vi "Set TWM Processing.vi"(4 "status ref (none)":refnum<vi>, 7 "Measurement properties":T1={"Measurement ID"=enum."1 signal, 1 ADC, 1 PJVS", "Description"="3 phase, 3 ADC, 1 PJVS", "Switching matrix M"=[], "Signal frequency  (Hz)"=50.0, "Maximal signal amplitude (V)"=0.0, "PRs (samples)"=0, "PRe (samples)"=0, "MRs (samples)"=0, "MRe (samples)"=0, "Set PJVS frequency (Hz)"=50.0, "PJVS reference voltages (1 period, V)"=[], "Requested PJVS frequency (Hz)"=50.0, "Requiested PJVS steps"=10, "Sampling f (Hz)"=7000.0, "Trigger mode"=enum."Trigger every MX switch", "Timing matrix (periods)"=[], "Record length (multiples of M)"=1, "Calculated"={"Triggers to next path (line of sequence)"=[], "Record samples"=0, "Sample indexes of switches"=[], "PRs (s)"=0.0, "PRe (s)"=0.0, "MRs (s)"=0.0, "MRe (s)"=0.0, "Trigger frequency  (Hz)"=50.0, "Measurement druation (s)"=0.0, "Samples per step"=0.0, "QPMX Sequence"=[], "PJVS segments frequency (Hz)"=50.0}, "No of required digitizers"=0, "No of required transducers"=0, "Transducer correction files"=[], "Digitizer correction file"=path "", "Algorithm"="TWM-PWRFFT", "plots_level"=1, "calc results"=FALSE, "Calculation mode"=enum."Standard"} {"Requested PJVS frequency (Hz)" format="%#_6p"; "plots_level" max=4 step=1; "Calculated"."Trigger frequency  (Hz)" format="%#_6p"; "Record length (multiples of M)" min=1 step=1; "PJVS reference voltages (1 period, V)" format="%.9g"}, 8 "error in":errorcluster, 11 "handle":i32) -> (0 "error out":errorcluster, 3 "handle out":i32)   [LabVIEW 2020]
doc: "Sets data processing in TWM. Sets algorithm and parameters."
uses:
  Type definitions/Measuement properties.ctl
  Type definitions/Measurement ID.ctl
  Type definitions/Trigger mode.ctl
  Type definitions/Calculation mode.ctl
  external libraries/TWM client/TWM Client Meas Setup.ctl
  external libraries/TWM client/TWM Client Meas Setup Trig.ctl
  external libraries/TWM client/TWM Client Processing Setup.ctl
  external libraries/TWM client/TWM Client.lvlib
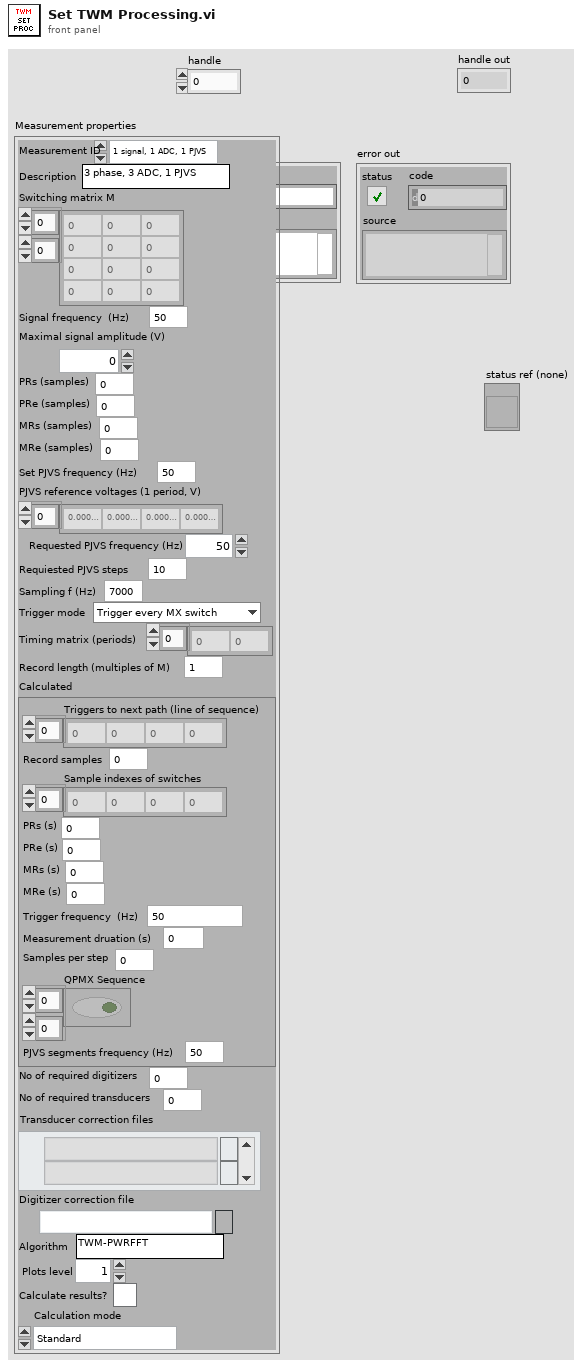
[diagram p1: front panel]
types:
  T1 = typedef "Measuement properties.ctl" = cluster{"Measurement ID":T2, "Description":string, "Switching matrix M":i32[][], "Signal frequency  (Hz)":dbl, "Maximal signal amplitude (V)":dbl, "PRs (samples)":u32, "PRe (samples)":u32, "MRs (samples)":u32, "MRe (samples)":u32, "Set PJVS frequency (Hz)":dbl, "PJVS reference voltages (1 period, V)":dbl[], "Requested PJVS frequency (Hz)":dbl, "Requiested PJVS steps":u32, "Sampling f (Hz)":dbl, "Trigger mode":T3, "Timing matrix (periods)":i32[], "Record length (multiples of M)":u32, "Calculated":cluster{"Triggers to next path (line of sequence)":u32[], "Record samples":u32, "Sample indexes of switches":u32[], "PRs (s)":dbl, "PRe (s)":dbl, "MRs (s)":dbl, "MRe (s)":dbl, "Trigger frequency  (Hz)":dbl, "Measurement druation (s)":dbl, "Samples per step":dbl, "QPMX Sequence":bool[][], "PJVS segments frequency (Hz)":dbl}, "No of required digitizers":u32, "No of required transducers":u32, "Transducer correction files":path[], "Digitizer correction file":path, "Algorithm":string, "plots_level":u32, "calc results":bool, "Calculation mode":T4}
  T2 = typedef "Measurement ID.ctl" = enum16{"Manual setup", "1 signal, 1 ADC, 1 PJVS", "1 phase (U, I), 1 ADC, 1 PJVS", "1 phase (U, I), 2 ADC, 1 PJVS, 4to1", "1 phase (U, I), 2 ADC, 1 PJVS, 2to1", "1 phase (U, I), 3 ADC, 1 PJVS", "3 phases (U1..3, I1..3), 3 ADC, 1 PJVS"}
  T3 = typedef "Trigger mode.ctl" = enum16{"Trigger every MX switch", "Trigger every sample"}
  T4 = typedef "Calculation mode.ctl" = enum16{"Standard", "Only synchronous power"}
  T5 = typedef "TWM Client.lvlib/TWM Client Processing Setup.ctl" = cluster{"calculate":i32, "all cycles at once":bool, "alg. ID":string, "unc mode":string, "mc cycles":i32, "timeout [s]":dbl, "loc [-]":dbl, "valid?":bool, "qwtb params":cluster{"name":string, "data":string[]}[]}
  T6 = typedef "TWM Client.lvlib/TWM Client Meas Setup Trig.ctl" = cluster{"valid?":bool, "coupling (T is DC)":bool, "slope (T is positive)":bool, "source (Immediate)":enum16{"Immediate", "Level", "External"}, "level [V]":dbl, "hysteresis [V]":dbl, "pre-trigger [%]":dbl}
  T7 = typedef "TWM Client.lvlib/TWM Client Meas Setup.ctl" = cluster{"smpl count":i32, "smpl rate [Hz]":dbl, "average":i32, "aperture [s]":dbl, "valid?":bool, "meas fld":path, "sub-records":i32, "ranges [Vpk]":dbl[], "smpl rate - fr [Hz]":dbl, "smpl rate - div":dbl, "smpl rate - mul":dbl, "offsets [V]":dbl[]}
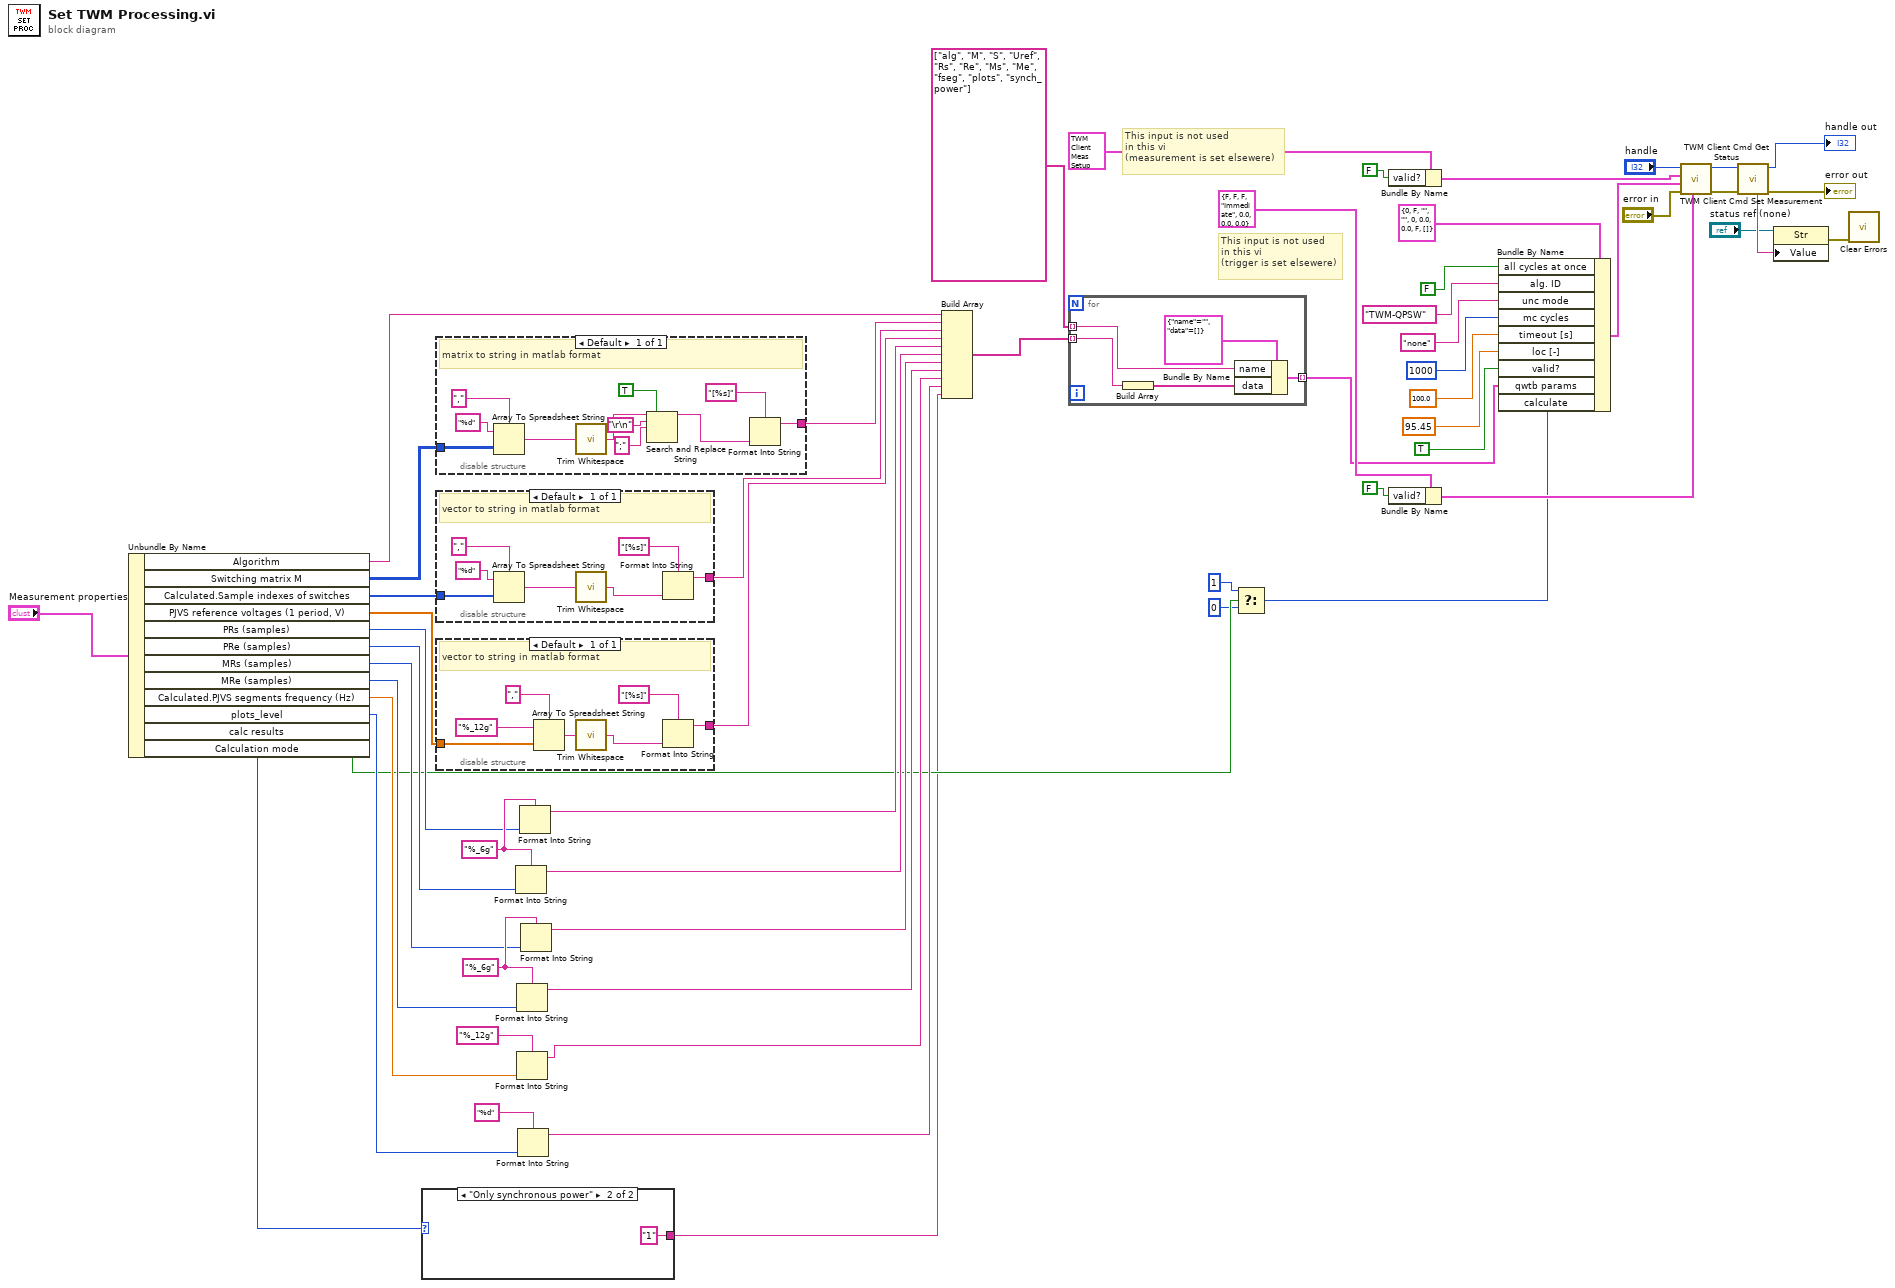
[diagram p0: block diagram]
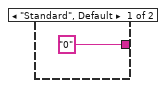
[diagram p2: hidden frame]
diagram:
  w26 = "%_6g" ("format string")
  w32 = "%_6g" ("format string")
  # "This input is not used\nin this vi\n(trigger is set elsewere)"
  # "This input is not used\nin this vi\n(measurement is set elsewere)"
  n1 = Unbundle By Name("Measurement properties") -> ("Algorithm"=w18:string, "Switching matrix M"=w38:i32[][], "Calculated.Sample indexes of switches"=w36:u32[], "PJVS reference voltages (1 period, V)"=w34:dbl[], "PRs (samples)"=w31:u32, "PRe (samples)"=w30:u32, "MRs (samples)"=w24:u32, "MRe (samples)"=w25:u32, "Calculated.PJVS segments frequency (Hz)"=w20:dbl, "plots_level"=w9:u32, "calc results"=w6:bool, "Calculation mode"=w2:T4)
  n2 = case shown="\"Only synchronous power\"" w2 {
    tunnel: ["0" ("format string") "1" ("format string")] -> w1
    frame "Standard", Default {
    }
    frame "Only synchronous power" {
    }
  }
  n3 = disable-structure shown="Default" {
    disable-tunnel: w38 -> [w61]
    disable-tunnel: [w60] -> w37
    frame Enabled {
      # "matrix to string in matlab format"
      n4 = Array To Spreadsheet String(delimiter (Tab)=",", array=w61, 3:"%d" ("format string")) -> (spreadsheet string=w65:string)
      n5 = call <vilib>:"Trim Whitespace.vi"("string"=w65) -> ("trimmed string"=w64:string)  [unwired: 1 in]
      n6 = Search and Replace String(replace all?=TRUE ("replace all? (F)"), input string=w64, search string="\r\n", replace string=";" ("replace string (\"\")")) -> (result string=w62:string)  [unwired: 4 in, 3 out]
      n7 = Format Into String(format string="[%s]", w62) -> (resulting string=w60:string)  [unwired: 2 in, 1 out]
    }
  }
  n8 = disable-structure shown="Default" {
    disable-tunnel: w36 -> [w74]
    disable-tunnel: [w71] -> w35
    frame Enabled {
      # "vector to string in matlab format"
      n9 = Array To Spreadsheet String(delimiter (Tab)=",", array=w74, 3:"%d" ("format string")) -> (spreadsheet string=w77:string)
      n10 = call <vilib>:"Trim Whitespace.vi"("string"=w77) -> ("trimmed string"=w72:string)  [unwired: 1 in]
      n11 = Format Into String(format string="[%s]", w72) -> (resulting string=w71:string)  [unwired: 2 in, 1 out]
    }
  }
  n12 = disable-structure shown="Default" {
    disable-tunnel: w34 -> [w79]
    disable-tunnel: [w78] -> w33
    frame Enabled {
      # "vector to string in matlab format"
      n13 = Array To Spreadsheet String(delimiter (Tab)=",", array=w79, 3:"%_12g" ("format string")) -> (spreadsheet string=w80:string)
      n14 = call <vilib>:"Trim Whitespace.vi"("string"=w80) -> ("trimmed string"=w84:string)  [unwired: 1 in]
      n15 = Format Into String(format string="[%s]", w84) -> (resulting string=w78:string)  [unwired: 2 in, 1 out]
    }
  }
  n16 = Format Into String(format string=w32, w30) -> (resulting string=w28:string)  [unwired: 2 in, 1 out]
  n17 = Format Into String(format string=w26, w25) -> (resulting string=w23:string)  [unwired: 2 in, 1 out]
  n18 = Format Into String(format string="%_12g", w20) -> (resulting string=w19:string)  [unwired: 2 in, 1 out]
  n19 = Format Into String(format string="%d", w9) -> (resulting string=w8:string)  [unwired: 2 in, 1 out]
  n20 = Format Into String(format string=w32, w31) -> (resulting string=w29:string)  [unwired: 2 in, 1 out]
  n21 = Format Into String(format string=w26, w24) -> (resulting string=w22:string)  [unwired: 2 in, 1 out]
  n22 = Build Array(w18, w37, w35, w33, w29, w28, w22, w23, w19, w8, w1) -> (w27:string[])
  n23 = for {
    tunnel: [w89] -> w43 mode=indexing
    tunnel: string[] ["alg", "M", "S", "Uref", "Rs", "Re", "Ms", "Me", "fseg", "plots", "synch_power"] -> [w88] mode=indexing
    tunnel: w27 -> [w87] mode=indexing
    n24 = Build Array(w87) -> (w86:string[])
    n25 = Bundle By Name(cluster=cluster{"name":string, "data":string[]} {"name"="", "data"=[]} ("Cluster"), "name"=w88, "data"=w86) -> (w89:cluster{"name":string, "data":string[]})
  }
  n26 = Select(t=1 ("calculate"), s=w6, f=0 ("calculate")) -> (s? t:f=w5:i32)
  n27 = Bundle By Name(cluster=T7 {"smpl count"=0, "smpl rate [Hz]"=0.0, "average"=0, "aperture [s]"=0.0, "valid?"=FALSE, "meas fld"=path "", "sub-records"=0, "ranges [Vpk]"=[], "smpl rate - fr [Hz]"=0.0, "smpl rate - div"=0.0, "smpl rate - mul"=0.0, "offsets [V]"=[]} ("meas"), "valid?"=FALSE) -> (w55:T7)
  n28 = Bundle By Name(cluster=T6 {"valid?"=FALSE, "coupling (T is DC)"=FALSE, "slope (T is positive)"=FALSE, "source (Immediate)"=enum."Immediate", "level [V]"=0.0, "hysteresis [V]"=0.0, "pre-trigger [%]"=0.0} ("Trigger"), "valid?"=FALSE) -> (w53:T6)
  n29 = Bundle By Name(cluster=T5 {"calculate"=0, "all cycles at once"=FALSE, "alg. ID"="", "unc mode"="", "mc cycles"=0, "timeout [s]"=0.0, "loc [-]"=0.0, "valid?"=FALSE, "qwtb params"=[]} ("processing"), "all cycles at once"=FALSE, "alg. ID"="TWM-QPSW", "unc mode"="none", "mc cycles"=1000, "timeout [s]"=100.0, "loc [-]"=95.45, "valid?"=TRUE, "qwtb params"=w43, "calculate"=w5) -> (w50:T5)
  n30 = call "TWM Client Cmd Set Measurement.vi"("Trigger"=w53, "error in"="error in", "processing"=w50, "meas"=w55, "handle"="handle") -> ("error out"=w16:errorcluster, "handle out"=w15:i32)  [unwired: 5 in]
  n31 = call "TWM Client Cmd Get Status.vi"("error in"=w16, "handle"=w15) -> ("error out"=→"error out":errorcluster, "handle out"=→"handle out":i32, "status string"=w12:string)  [unwired: 5 in, 2 out]
  n32 = property class="Str"(reference="status ref (none)", "Value"=w12) -> (error out=w17:errorcluster)  [unwired: 1 in, 1 out]
  n33 = call <vilib>:"Clear Errors.vi"("error in (no error)"=w17) -> ()  [unwired: 5 in, 2 out]
